vi "Get Double By Name.vi"(0 "name":string, 2 "Analog Values":T1) -> (7 "result":dbl, 9 "found?":bool)   [LabVIEW 2013]
uses:
  Hardware Interface/DblArrayWithName.ctl
  Hardware Interface/Hardware Interface.lvclass
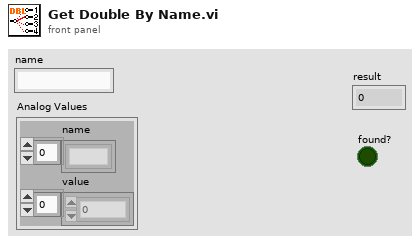
[diagram p1: front panel]
types:
  T1 = typedef "Hardware Interface.lvclass/DblArrayWithName.ctl" = cluster{"name":string[], "value":dbl[]}
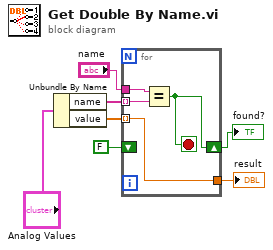
[diagram p0: block diagram]
diagram:
  n1 = Unbundle By Name("Analog Values") -> ("name"=w7:string[], "value"=w6:dbl[])
  n2 = for {
    tunnel: w7 -> [w9] mode=indexing
    tunnel: w6 -> [w11] mode=indexing
    tunnel: [w11] -> w1
    tunnel: "name" -> [w10]
    shift-right: [w8] -> w3
    shift-left: FALSE -> [_]
    stop <- w8 stop-if-true
    n3 = Equal?(x=w10, y=w9) -> (x = y?=w8:bool)
  }
  "found?" <- w3
  "result" <- w1
